vi "Read WCM_limits.vi"(8 "error in (no error)":errorcluster, 11 "Experiment in":refnum<class "Experiment.lvclass">) -> (0 "error out":errorcluster, 2 "WCM_limits":T1, 3 "Experiment out":refnum<class "Experiment.lvclass">)   [LabVIEW 2019, in "Experiment.lvclass"]
uses:
  Experiment.lvclass
  dependecies/ControlsVIs/Clusters-def/Def_WCM_limits.ctl
  Experiment.lvclass/Experiment.ctl
  Oscilloscope/Oscilloscope.lvclass
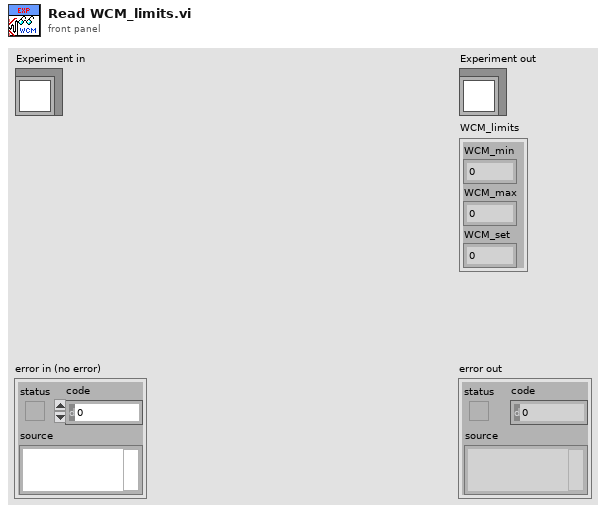
[diagram p1: front panel]
types:
  T1 = typedef "Oscilloscope.lvclass/Def_WCM_limits.ctl" = cluster{"WCM_min":dbl, "WCM_max":dbl, "WCM_set":dbl}
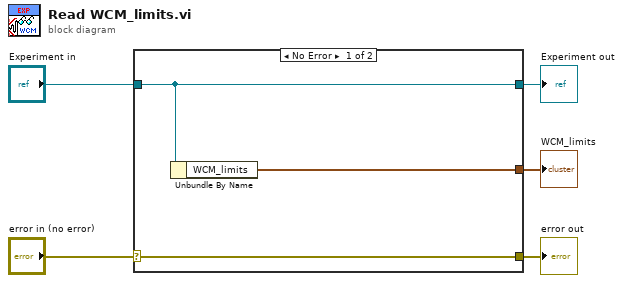
[diagram p0: block diagram]
diagram:
  n1 = case shown="No Error" "error in (no error)" {
    selector: "error in (no error)" -> [w8 w9]
    tunnel: [w8 w9] -> w4
    tunnel: [w7 w10] -> w2
    tunnel: "Experiment in" -> [w7 w10]
    tunnel: [w6 _] -> w1
    frame No Error {
      n2 = Unbundle By Name(w7) -> ("WCM_limits"=w6:T1)
    }
    frame Error {
    }
  }
  "error out" <- w4
  "Experiment out" <- w2
  "WCM_limits" <- w1
